vi "RT CAN Transceiver.vi"() -> ()   [LabVIEW 2024]
uses:
  Shared Modules/CAN Commands Interpreter/CAN Frame Data.ctl
  Shared Modules/CAN Commands Interpreter/Command Values.ctl
  Shared Modules/CAN Commands Interpreter/XNET Session Settings.ctl
  Shared Modules/CAN Commands Interpreter/Target Sessions - Initialize Output Session.vi
  Shared Modules/CAN Commands Interpreter/Target Sessions - Initialize Input Session.vi
  Shared Modules/CAN Commands Interpreter/Target Sessions - Stop Session.vi
  Shared Modules/CAN Commands Interpreter/Target Sessions - Start Session.vi
  Shared Modules/CAN Commands Interpreter/CAN Commands.lvlib
panel:
  in  "Tab Control":enum32{"Sessions", "Monitor", "Errors"}(tab)
  in  "ECU Sessions":T1[][](array[typedef])=[[{"Interface"="CAN1", "Frame List"=["Tester_Requests\nCAN Dataframes"], "Session ID"="", "Session Name"="ECU - Read Tester Requests"}, {"Interface"="CAN1", "Frame List"=["ECU_Responses\nCAN Dataframes"], "Session ID"="", "Session Name"="ECU - Write ECU Responses"}, {"Interface"="CAN1", "Frame List"=["HeartBit\nCAN Dataframes"], "Session ID"="", "Session Name"="ECU - Write Hertbit"}], [{"Interface"="CAN1", "Frame List"=["Crank_Angle\nCAN Dataframes"], "Session ID"="", "Session Name"="ECU - Write Crank Angle"}, {"Interface"="CAN1", "Frame List"=["Throttle\nCAN Dataframes"], "Session ID"="", "Session Name"="ECU - Write Throttle"}, {"Interface"="", "Frame List"=[], "Session ID"="", "Session Name"=""}]]
  out "XNET Data":T2[](array[typedef]) {"ID" format="%01x"; "Payload" format="%02x"}
  in  "STOP":bool
  in  "Send command to Tester":bool
  in  "Command":T3={"Command"="Voltage Out Enabled", "Value"=0.0}
  out "Working Mode":T4(ring)
  out "Target Connected":bool
  out "Target Found":bool
  out "Read Error":errorcluster
  out "Write Error":errorcluster
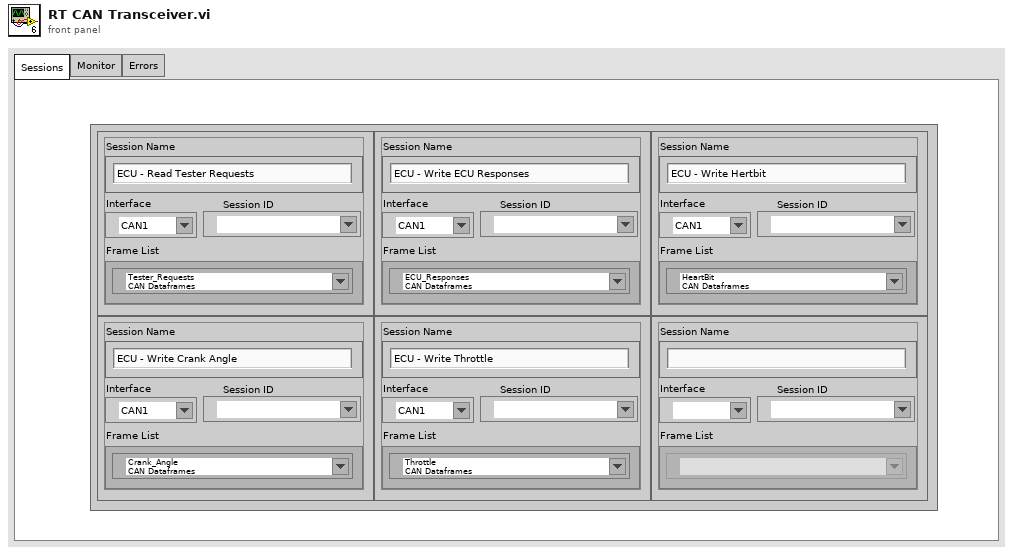
[diagram p1: front panel]
types:
  T1 = typedef "CAN Commands.lvlib/XNET Session Settings.ctl" = cluster{"Interface":refnum<k21>, "Frame List":refnum<k21>[], "Session ID":refnum<k21>, "Session Name":string}
  T2 = typedef "CAN Commands.lvlib/CAN Frame Data.ctl" = cluster{"Command":string, "XNET Frame":refnum<k21>, "Payload":u8[], "ID":u32, "Time Stamp":timestamp}
  T3 = typedef "CAN Commands.lvlib/Command Values.ctl" = cluster{"Command":string, "Value":dbl}
  T4 = enum16{"Init", "Wait For Tester", "Set Normal Mode", "Run Normal Mode", "Set Manufacturing Mode", "Run Manufacturing Mode", "End"}
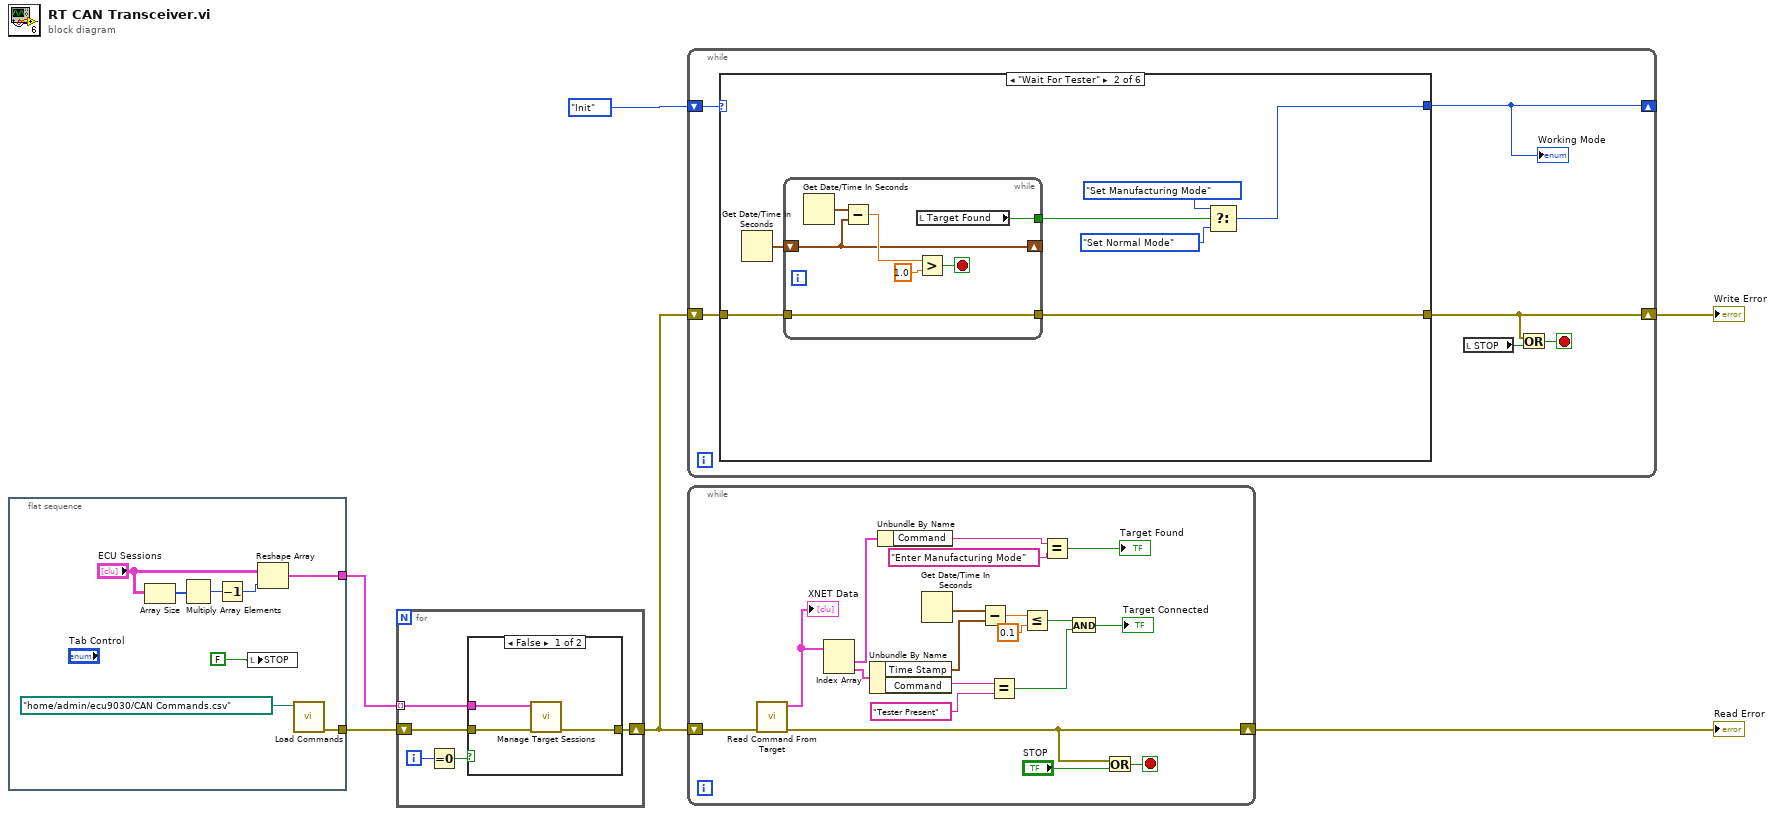
[diagram p0: block diagram]
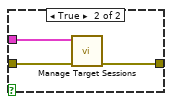
[diagram p2: hidden frame]
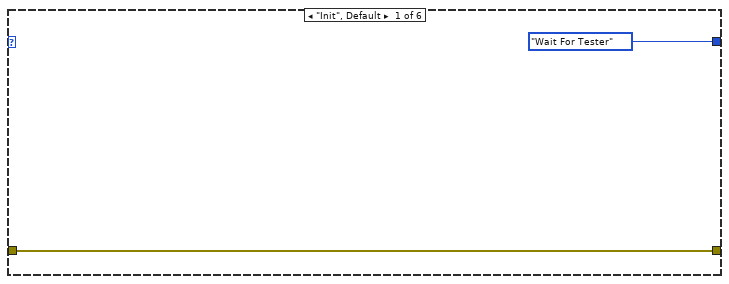
[diagram p3: hidden frame]
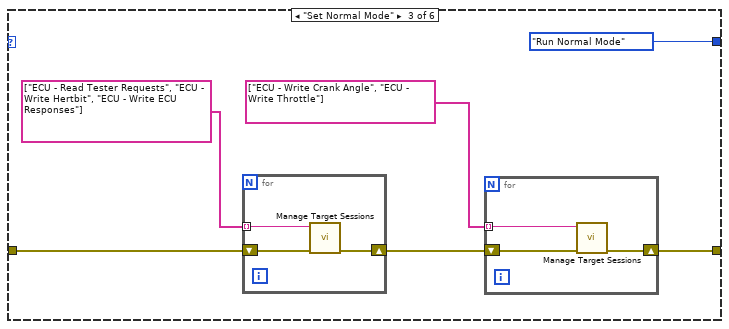
[diagram p4: hidden frame]
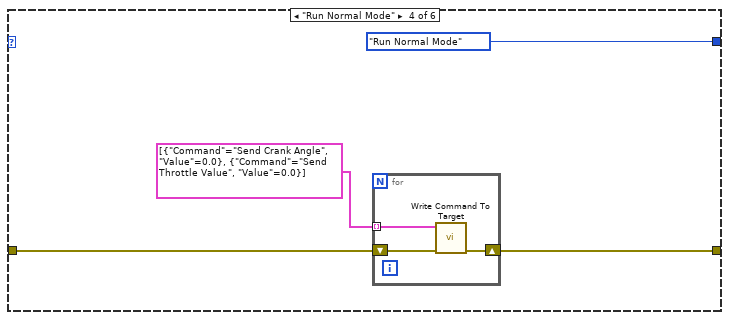
[diagram p5: hidden frame]
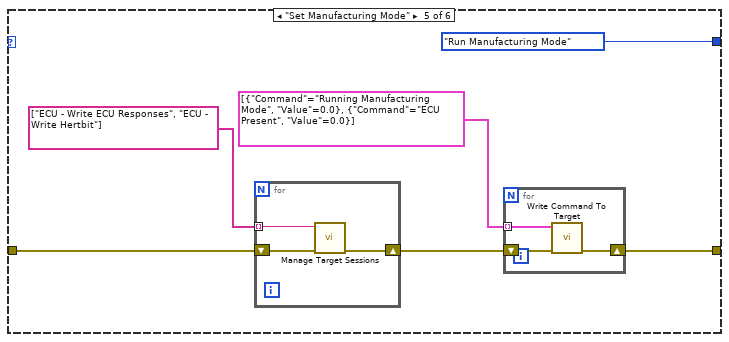
[diagram p6: hidden frame]
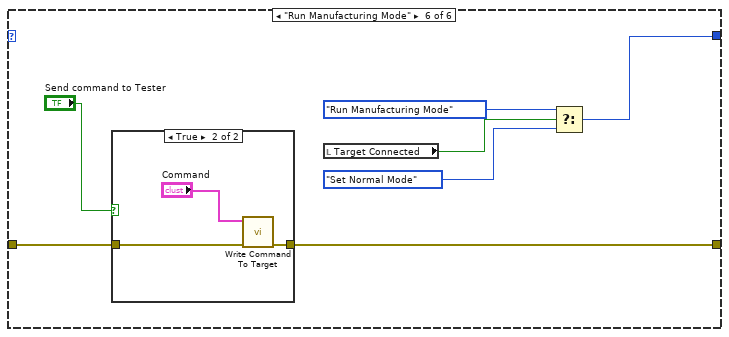
[diagram p7: hidden frame]
diagram:
  n1 = flat-sequence {
    tunnel: [w14] -> w6
    tunnel: [w7] -> w1
    frame #0 {
      n2 = Array Size(array="ECU Sessions") -> (size(s)=w8:i32[])
      n3 = Multiply Array Elements(1:w8) -> (0:w9:i32)
      n4 = Decrement(x=w9) -> (x-1=w11:i32)
      n5 = local write "STOP"(FALSE ("STOP")) -> ()
      n6 = Reshape Array("ECU Sessions", w11) -> (w7:T1[])
      n7 = call "Load Commands.vi"("Commands File (CSV)"=path "/home/admin/ecu9030/CAN Commands.csv") -> ("error out"=w14:errorcluster)  [unwired: 10 in]
    }
  }
  n8 = for {
    shift-right: [w19] -> w4
    shift-left: w6 -> [w18]
    tunnel: w1 -> [w15] mode=indexing
    i -> [w16]
    n9 = Equal To 0?(x=w16) -> (x = 0?=w17:bool)
    n10 = case shown="False" w17 {
      tunnel: [w21 w25] -> w19
      tunnel: w18 -> [w22 w24]
      tunnel: w15 -> [w20 w23]
      frame False {
        n11 = call-poly "Manage Target Sessions.vi"("error in"=w22, "XNET Session Resouces"=w20) -> ("error out"=w21:errorcluster)  [unwired: 9 in]
      }
      frame True {
        n12 = call-poly "Manage Target Sessions.vi"("error in"=w24, "XNET Session Resouces"=w23) -> ("error out"=w25:errorcluster)  [unwired: 9 in]
      }
    }
  }
  n13 = while {
    shift-right: [w27] -> w3
    shift-left: w4 -> [w28]
    shift-right: [w26] -> _
    shift-left: T4."Init" -> [w29]
    stop <- w30 stop-if-true
    n14 = case shown="\"Wait For Tester\"" w29 {
      tunnel: [T4."Wait For Tester" w35 T4."Run Normal Mode" T4."Run Normal Mode" T4."Run Manufacturing Mode" w79] -> w26
      tunnel: w28 -> [w32 w39 w50 w62 w70 w85]
      tunnel: [w32 w38 w52 w61 w68 w84] -> w27
      frame "Init", Default {
      }
      frame "Wait For Tester" {
        n15 = Get Date/Time In Seconds() -> (seconds since 1Jan1904=w40:timestamp)
        n16 = while {
          shift-right: [w44] -> _
          shift-left: w40 -> [w44]
          tunnel: [w42] -> w34
          tunnel: w39 -> [w41]
          tunnel: [w41] -> w38
          stop <- w43 stop-if-true
          n17 = Get Date/Time In Seconds() -> (seconds since 1Jan1904=w47:timestamp)
          n18 = Subtract(x=w47, y=w44) -> (x-y=w45:dbl)
          n19 = local read "Target Found"() -> (w42:bool)
          n20 = Greater?(x=w45, y=1.0) -> (0:w43:bool)
        }
        n21 = Select(t=T4."Set Manufacturing Mode", s=w34, f=T4."Set Normal Mode") -> (s? t:f=w35:T4)
      }
      frame "Set Normal Mode" {
        n22 = for {
          shift-right: [w56] -> w49
          shift-left: w50 -> [w55]
          tunnel: string[] ["ECU - Read Tester Requests", "ECU - Write Hertbit", "ECU - Write ECU Responses"] -> [w54] mode=indexing
          n23 = call-poly "Manage Target Sessions.vi"("error in"=w55, "Session Name"=w54) -> ("error out"=w56:errorcluster)  [unwired: 9 in]
        }
        n24 = for {
          tunnel: string[] ["ECU - Write Crank Angle", "ECU - Write Throttle"] -> [w59] mode=indexing
          shift-right: [w58] -> w52
          shift-left: w49 -> [w57]
          n25 = call-poly "Manage Target Sessions.vi"("error in"=w57, "Session Name"=w59) -> ("error out"=w58:errorcluster)  [unwired: 9 in]
        }
      }
      frame "Run Normal Mode" {
        n26 = for {
          tunnel: T3[] [{"Command"="Send Crank Angle", "Value"=0.0}, {"Command"="Send Throttle Value", "Value"=0.0}] -> [w66] mode=indexing
          shift-right: [w64] -> w61
          shift-left: w62 -> [w65]
          n27 = call "Write Command To Target.vi"("error out"=w65, "Command"=w66) -> ("error out"=w64:errorcluster)  [unwired: 9 in]
        }
      }
      frame "Set Manufacturing Mode" {
        n28 = for {
          tunnel: string[] ["ECU - Write ECU Responses", "ECU - Write Hertbit"] -> [w78] mode=indexing
          shift-right: [w77] -> w72
          shift-left: w70 -> [w76]
          n29 = call-poly "Manage Target Sessions.vi"("error in"=w76, "Session Name"=w78) -> ("error out"=w77:errorcluster)  [unwired: 9 in]
        }
        n30 = for {
          shift-right: [w74] -> w68
          shift-left: w72 -> [w75]
          tunnel: T3[] [{"Command"="Running Manufacturing Mode", "Value"=0.0}, {"Command"="ECU Present", "Value"=0.0}] -> [w73] mode=indexing
          n31 = call "Write Command To Target.vi"("error out"=w75, "Command"=w73) -> ("error out"=w74:errorcluster)  [unwired: 9 in]
        }
      }
      frame "Run Manufacturing Mode" {
        n32 = case shown="True" "Send command to Tester" {
          tunnel: w85 -> [w86 w89]
          tunnel: [w86 w88] -> w84
          frame False {
          }
          frame True {
            n33 = call "Write Command To Target.vi"("error out"=w89, "Command"="Command") -> ("error out"=w88:errorcluster)  [unwired: 9 in]
          }
        }
        n34 = local read "Target Connected"() -> (w82:bool)
        n35 = Select(t=T4."Run Manufacturing Mode", s=w82, f=T4."Set Normal Mode") -> (s? t:f=w79:T4)
      }
    }
    "Working Mode" <- w26
    n36 = local read "STOP"() -> (w31:bool)
    n37 = Or(x=w27, y=w31) -> (x .or. y?=w30:bool)
  }
  "Write Error" <- w3
  n38 = while {
    shift-right: [w105] -> w5
    shift-left: w4 -> [w108]
    stop <- w106 stop-if-true
    n39 = call "Read Command From Target.vi"("error in"=w108) -> ("error out"=w105:errorcluster, "XNET Data"=w103:T2[])  [unwired: 7 in, 2 out]
    "XNET Data" <- w103
    n40 = Index Array(array=w103) -> (element #1=w94:T2, element #2=w102:T2)  [unwired: 2 in]
    n41 = Unbundle By Name(w102) -> ("Time Stamp"=w101:timestamp, "Command"=w97:string)
    n42 = Unbundle By Name(w94) -> ("Command"=w93:string)
    n43 = Get Date/Time In Seconds() -> (seconds since 1Jan1904=w104:timestamp)
    n44 = Subtract(x=w104, y=w101) -> (x-y=w100:dbl)
    n45 = Equal?(x=w97, y="Tester Present") -> (x = y?=w95:bool)
    n46 = Less Or Equal?(x=w100, y=0.1) -> (x <= y?=w98:bool)
    n47 = Equal?(x=w93, y="Enter Manufacturing Mode") -> (x = y?=→"Target Found":bool)
    n48 = And(x=w98, y=w95) -> (x .and. y?=→"Target Connected":bool)
    n49 = Or(x=w105, y="STOP") -> (x .or. y?=w106:bool)
  }
  "Read Error" <- w5
